vi "NicmosProcessData.vi"(2 "Index":i32, 3 "Data In":T2, 9 "error out":errorcluster caption="error in (no error)") -> (0 "Data Out":T1, 6 "error in (no error)":errorcluster caption="error out")   [LabVIEW 2009]
uses:
  Controls/NICMOS.RAW.ctl
  Controls/NICMOS.DATA.ctl
  NicmosGlobal.vi
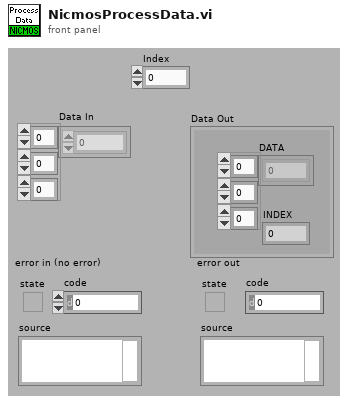
[diagram p1: front panel]
types:
  T1 = typedef "NICMOS.DATA.ctl" = cluster{"DATA":i32[][][], "INDEX":i32}
  T2 = typedef "NICMOS.RAW.ctl" = u16[][][]
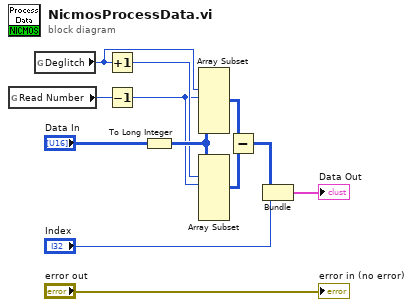
[diagram p0: block diagram]
diagram:
  n1 = global read "NicmosGlobal.vi" "Read Number"() -> (w12:i32)
  n2 = global read "NicmosGlobal.vi" "Deglitch"() -> (w7:i32)
  n3 = Increment(x=w7) -> (x+1=w9:i32)
  n4 = Decrement(x=w12) -> (x-1=w8:i32)
  n5 = To Long Integer(number="Data In") -> (32bit integer=w10:i32[][][])
  n6 = Array Subset(array=w10, index (dim 0)=w7, length (dim 0)=w8) -> (w11:i32[][][])  [unwired: 4 in]
  n7 = Array Subset(array=w10, index (dim 0)=w9, length (dim 0)=w8) -> (w6:i32[][][])  [unwired: 4 in]
  n8 = Subtract(x=w11, y=w6) -> (x-y=w3:i32[][][])
  n9 = Bundle(w3, "Index"="Index") -> (→"Data Out":cluster{i32[][][], "Index":i32})  [unwired: 1 in]
  "error in (no error)" <- "error out"
